vi "XLP80_FGlob_InitFuncGlobs.vi"(8 "err in":errorcluster caption="error") -> (0 "err out":errorcluster caption="error")   [LabVIEW 2021]
uses:
  XLP80_FGLob_TDefEnumCalcAnalogItems.ctl
  XLP80_FGLob_TDefEnumCalcBoolItems.ctl
  1886_FGlob_TDefs_Enum_FGlobItems.ctl
  XLP80_Globals/XLP80_Globals_Status.vi
  XLP80_Globals/Globals_Settings_XLP80.vi
  XLP80_General_Libs/WL_Libs_V14.25/WL_Chart_V17.01_mod.llb/WL_Chart_Globals.vi
panel:
  in  "CalculatedBool_Items":T1
  in  "CalculatedAnalog_Items":T2
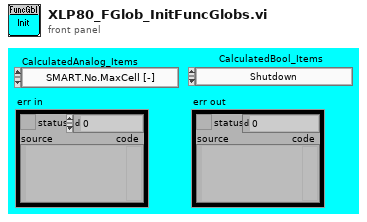
[diagram p1: front panel]
types:
  T1 = typedef "XLP80_FGLob_TDefEnumCalcBoolItems.ctl" = enum8{"Shutdown", "Alarm", "but_NotAus"}
  T2 = typedef "XLP80_FGLob_TDefEnumCalcAnalogItems.ctl" = enum8{"SMART.No.MaxCell [-]", "SMART.No.MinCell [-]", "SMART.U.S.AveCell [V]", "SMART.U.S.CVM [V]", "SMART.U.S.MaxCell [V]", "SMART.U.S.MinCell [V]"}
  T3 = typedef "1886_FGlob_TDefs_Enum_FGlobItems.ctl" = enum16{"Put one", "Put all", "Recall one", "Recall all"}
  T4 = typedef "XLP80_Action_TDefEnumControl.ctl" = enum16{"Testmode_A", "Testmode_B"}
  T5 = cluster{"Initialize (F)":bool, "# channels":i32, "Puffergröße":i32}
  T6 = cluster{"Signal Name":string[], "Description":string[], "Unit":string[], "Default":dbl[], "Min":dbl[], "Max":dbl[], "Preconditions":bool[], "HV & Software":bool[], "Basis Funktion":bool[], "Power Management":bool[], "OperationMode":bool[], "Shutdown":bool[], "Alarm":bool[], "LogEnable":bool[]}
  T7 = cluster{"Signal Name":string[], "Description":string[], "Unit":string[], "Min":dbl[], "Max":dbl[], "HV & Software":bool[], "Basis Funktion":bool[], "Power Management":bool[], "OperationMode":bool[], "Shutdown":bool[], "Alarm":bool[], "LogEnable":bool[]}
  T8 = cluster{"LineStyle":u8[], "LineWidth":u8[], "LineColor":u32[], "SelectedPlot":i32[], "Scales":u16[], "Enabled":bool[]}
  T9 = cluster{"Signal Name":string[], "Description":string[], "Unit":string[], "Default":dbl[], "Min":dbl[], "Max":dbl[], "TestmodeA":bool[], "LogEnable":bool[]}
  T10 = typedef "KH_DAQ_TypeDefs_Cluster AO.ctl" = cluster{"Signal Name":string[], "Description":string[], "Phys Unit":string[], "Messbereich":T11[], "Chan":u16[], "Phys Min":sgl[], "Phys Max":sgl[], "Offset":sgl[], "Nr":u16[], "SensorType 2":T12[], "Bereich":T13[], "Default":sgl[]}
  T11 = typedef "KH_DAQ_TypeDefs_Messbereich.ctl" = enum16{"-10V ... +10V", "0V ... +10V", "+2V ... +10V", "0V ... +5V", "+1V ... +5V", "-1V ... +1V", "-500mV ... +500mV", "-100mV ... +100mV", "-50mV ... +50mV", "0mA ... +20mA", "+4mA ... +20mA", "-20mA ... +20mA", "0 Ohm ... 100 Ohm", "0 Ohm ... 400 Ohm", "0 Ohm ... 2000 Ohm", "0 Ohm ... 4000 Ohm", "-200°C ... 150°C PT100", "-200°C ... 150°C PT200", "-200°C ... 150°C PT500", "-200°C ... 150°C PT1000", "-60°C ... 150°C Ni100", "-60°C ... 150°C Ni1000", "-200°C ... 850°C PT100", "-200°C ... 850°C PT200", "-200°C ... 850°C PT500", "-200°C ... 850°C PT1000", "-50°C ... 250°C Ni100", "-50°C ... 250° Ni 1000"}
  T12 = typedef "KH EthernetIPConfig TypeDefs ModuleTyp.ctl" = enum16{"TBEN-S2-4AI", "TBEN-S1-8DXP", "TBEN-S2-2RFID-4DXP", "TBEN-S2-4AO", "TBEN-S2-4IOL"}
  T13 = typedef "KH_DAQ_TypeDefs_Bereich.ctl" = enum16{"Standard", "extended Range", "NE43", ""}
  T14 = typedef "KH_DAQ_TypeDefs_Cluster AI.ctl" = cluster{"Signal Name":string[], "Description":string[], "Phys Unit":string[], "Messbereich":T11[], "Chan":u16[], "Phys Min":sgl[], "Phys Max":sgl[], "Offset":sgl[], "Nr":u16[], "SensorType 2":T12[], "Bereich":T13[]}
  T15 = typedef "KH_DAQ_TURCK_TypeDefs_Cluster DI.ctl" = cluster{"Signal Name":string[], "Description":string[], "Chan":u16[], "Inv":bool[], "Nr":u16[], "SensorType":T12[]}
  T16 = typedef "KH_DAQ_TURCK_TypeDefs_Cluster DO.ctl" = cluster{"Def":bool[], "Signal Name":string[], "Description":string[], "Chan":u16[], "Inv":bool[], "Nr":u16[], "SensorType":T12[]}
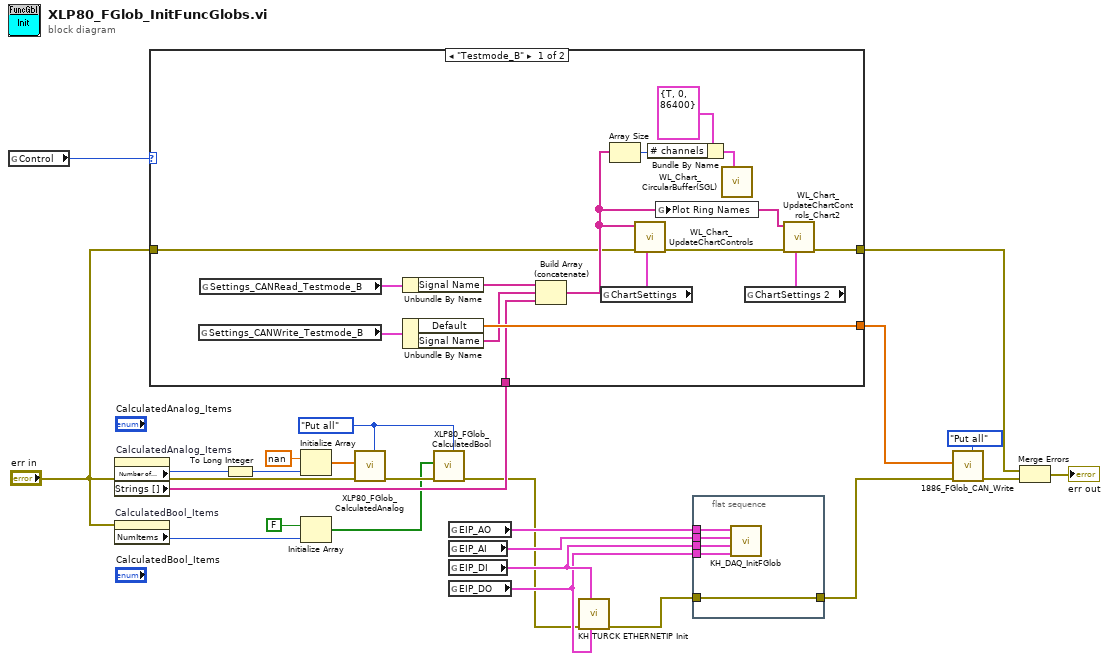
[diagram p0: block diagram]
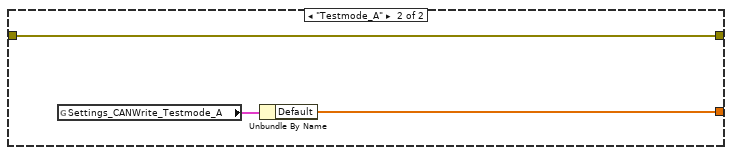
[diagram p2: hidden frame]
diagram:
  w4 = 1886_FGlob_TDefs_Enum_FGlobItems."Put all" ("Function (Recall One)")
  n1 = global read "XLP80_Globals_Status.vi" "Control"() -> (w18:T4)
  n2 = property on="CalculatedAnalog_Items" class="Enum (strict)"() -> ("Number of Items"=w22:u32, "Strings []"=w16:string[])  [unwired: 2 in, 2 out]
  n3 = property on="CalculatedBool_Items" class="Enum (strict)"(error in="err in") -> ("NumItems"=w3:u32)  [unwired: 1 in, 2 out]
  n4 = case shown="\"Testmode_B\"" w18 {
    tunnel: [w38 w41] -> w17
    tunnel: w16 -> [w34 _]
    tunnel: "err in" -> [w27 w40]
    tunnel: [w26 w40] -> w14
    frame "Testmode_B" {
      n5 = global read "Globals_Settings_XLP80.vi" "Settings_CANWrite_Testmode_B"() -> (w39:T6)
      n6 = global read "Globals_Settings_XLP80.vi" "Settings_CANRead_Testmode_B"() -> (w37:T7)
      n7 = Unbundle By Name(w37) -> ("Signal Name"=w36:string[])
      n8 = Unbundle By Name(w39) -> ("Default"=w38:dbl[], "Signal Name"=w35:string[])
      n9 = Build Array (concatenate)(w36, w35, w34) -> (w29:string[])
      n10 = global read "Globals_Settings_XLP80.vi" "ChartSettings"() -> (w28:T8)
      n11 = Array Size(array=w29) -> (size(s)=w32:i32)
      n12 = call "WL_Chart_UpdateChartControls.vi"("ChartSettings"=w28, "err in"=w27, "PlotNames"=w29) -> ("err out"=w33:errorcluster)  [unwired: 8 in]
      n13 = Bundle By Name(cluster=T5 {"Initialize (F)"=TRUE, "# channels"=0, "Puffergröße"=86400} ("Init"), "# channels"=w32) -> (w31:T5)
      n14 = global write "WL_Chart_Globals.vi" "Plot Ring Names"(w29) -> ()
      n15 = call "WL_Chart_CircularBuffer(SGL).vi"("Init"=w31) -> ()  [unwired: 5 in, 6 out]
      n16 = global read "Globals_Settings_XLP80.vi" "ChartSettings 2"() -> (w25:T8)
      n17 = call "WL_Chart_UpdateChartControls_Chart2.vi"("ChartSettings 2"=w25, "err in"=w33, "PlotNames"=w29) -> ("err out"=w26:errorcluster)  [unwired: 8 in]
    }
    frame "Testmode_A" {
      n18 = global read "Globals_Settings_XLP80.vi" "Settings_CANWrite_Testmode_A"() -> (w42:T9)
      n19 = Unbundle By Name(w42) -> ("Default"=w41:dbl[])
    }
  }
  n20 = To Long Integer(number=w22) -> (32bit integer=w21:i32)
  n21 = Initialize Array(sgl nan ("element"), w21) -> (w23:sgl[])
  n22 = Initialize Array(FALSE, w3) -> (w1:bool[])
  n23 = call "XLP80_FGlob_CalculatedAnalog.vi"("Function (Recall One)"=w4, "err in"="err in", "Calc Values IN"=w23) -> ("err out"=w6:errorcluster)  [unwired: 6 in, 2 out]
  n24 = call "XLP80_FGlob_CalculatedBool.vi"("Function (Recall One)"=w4, "err in"=w6, "Calc Values IN"=w1) -> ("err out"=w5:errorcluster)  [unwired: 6 in, 2 out]
  n25 = global read "Globals_Settings_XLP80.vi" "EIP_AO"() -> (w11:T10)
  n26 = global read "Globals_Settings_XLP80.vi" "EIP_AI"() -> (w10:T14)
  n27 = global read "Globals_Settings_XLP80.vi" "EIP_DI"() -> (w9:T15)
  n28 = global read "Globals_Settings_XLP80.vi" "EIP_DO"() -> (w8:T16)
  n29 = call "KH TURCK ETHERNETIP Init.vi"("EIP_DO"=w8, "EIP_DI"=w9, "err in"=w5) -> ("err out"=w13:errorcluster)  [unwired: 8 in]
  n30 = flat-sequence {
    tunnel: w11 -> [w47]
    tunnel: w10 -> [w46]
    tunnel: w9 -> [w45]
    tunnel: w8 -> [w44]
    tunnel: w13 -> [w43]
    tunnel: [w43] -> w12
    frame #0 {
      n31 = call "KH_DAQ_InitFGlob.vi"("EIP_DO"=w44, "EIP_DI"=w45, "EIP_AI"=w46, "EIP_AO"=w47) -> ()  [unwired: 8 in]
    }
  }
  n32 = call "1886_FGlob_CAN_Write.vi"("Function (Recall One)"=1886_FGlob_TDefs_Enum_FGlobItems."Put all", "err in"=w12, "AO Values IN"=w17) -> ("err out"=w19:errorcluster)  [unwired: 6 in, 2 out]
  n33 = Merge Errors(w14, w19) -> (→"err out":errorcluster)
